vi "Read Time Out (SubVI).vi"(8 "error in (no error)":errorcluster, 9 "Time Out (ms)":u32=1000, 11 "DIO Reference":T1) -> (0 "Error Out":errorcluster, 3 "DIO Ref Out":T1)   [LabVIEW 2013]
uses:
  <vilib>/myRIO/Instrument Drivers/Onboard IO/DIO/typedefs/DIO Reference.ctl
  <vilib>/myRIO/Common/Instrument Driver Framework/Utilities/typedefs/myRIO Generic Hardware Reference.ctl
  <vilib>/myRIO/Common/Instrument Driver Framework/Utilities/typedefs/Hardware Version Enum.ctl
  <vilib>/myRIO/Common/Instrument Driver Framework/Utilities/typedefs/myRIO v1.0 Reference.ctl
  <vilib>/myRIO/Common/Instrument Driver Framework/Utilities/typedefs/Generic FPGA Reference.ctl
  <vilib>/myRIO/Common/Instrument Driver Framework/myRIO v1.0/DIO/typedefs/DIO Channels List.ctl
  <vilib>/myRIO/Common/Instrument Driver Framework/myRIO v1.0/DIO/typedefs/DIO Channels Enum.ctl
  TimeOutError.ctl
  <vilib>/Utility/error.llb/Error Cluster From Error Code.vi
  <vilib>/myRIO/Common/Instrument Driver Framework/myRIO v1.0/DIO/vis/myRIO v1.0 Read DIO.vi
  <vilib>/myRIO/Instrument Drivers/Onboard IO/DIO/DIO.lvlib
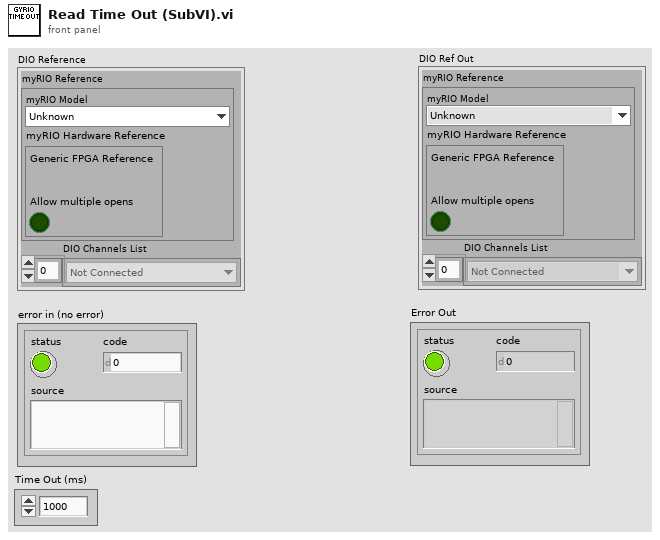
[diagram p1: front panel]
types:
  T1 = typedef "DIO.lvlib/DIO Reference.ctl" = cluster{"myRIO Reference":T2, "DIO Channels List":T6}
  T2 = typedef "myRIO Generic Hardware Reference.ctl" = cluster{"myRIO Model":T3, "myRIO Hardware Reference":T4}
  T3 = typedef "Hardware Version Enum.ctl" = enum16{"Unknown", "myRIO-1900", "myRIO-1950"}
  T4 = typedef "myRIO v1.0 Reference.ctl" = cluster{"Generic FPGA Reference":T5, "Allow multiple opens":bool}
  T5 = typedef "Generic FPGA Reference.ctl" = refnum<k20>
  T6 = typedef "DIO Channels List.ctl" = T7[]
  T7 = typedef "DIO Channels Enum.ctl" = enum16{"Not Connected", "C/DIO0", "C/DIO1", "C/DIO2", "C/DIO3", "C/DIO4", "C/DIO5", "C/DIO6", "C/DIO7", "A/DIO0", "A/DIO1", "A/DIO2", "A/DIO3", "A/DIO4", "A/DIO5", "A/DIO6", "A/DIO7", "A/DIO8", "A/DIO9", "A/DIO10", "A/DIO11", "A/DIO12", "A/DIO13", "A/DIO14", "A/DIO15", "B/DIO0", "B/DIO1", "B/DIO2", "B/DIO3", "B/DIO4", "B/DIO5", "B/DIO6", "B/DIO7", "B/DIO8", "B/DIO9", "B/DIO10", "B/DIO11", "B/DIO12", "B/DIO13", "B/DIO14", "B/DIO15", "LED0", "LED1", "LED2", "LED3", "Button0"}
  T8 = typedef "TimeOutError.ctl" = errorcluster
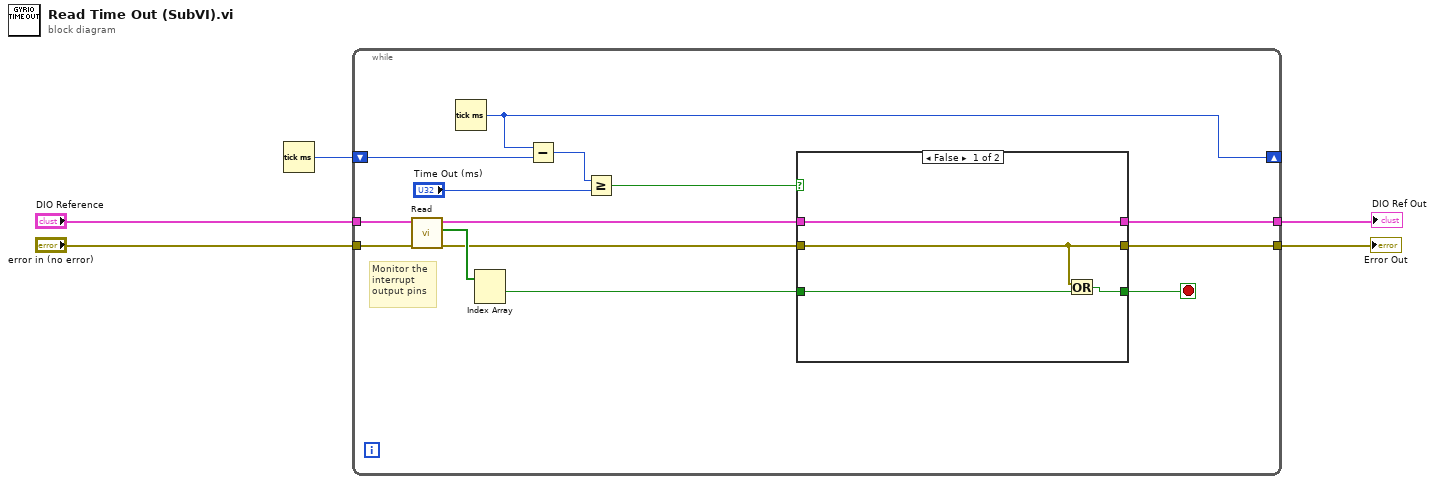
[diagram p0: block diagram]
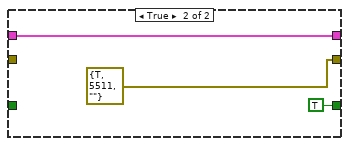
[diagram p2: hidden frame]
diagram:
  n1 = Tick Count (ms)() -> (millisecond timer value=w1:u32)
  n2 = while {
    tunnel: "error in (no error)" -> [w18]
    tunnel: "DIO Reference" -> [w17]
    tunnel: [w6] -> w2
    tunnel: [w7] -> w3
    shift-right: [w10] -> _
    shift-left: w1 -> [w13]
    stop <- w15 stop-if-true
    # "Monitor the\ninterrupt\noutput pins"
    n3 = call <vilib>:"Read.vi"("error in (no error)"=w18, "DIO Ref In"=w17) -> ("error out"=w14:errorcluster, "Values"=w19:bool[], "DIO Ref Out"=w8:T1)  [unwired: 7 in]
    n4 = Tick Count (ms)() -> (millisecond timer value=w10:u32)
    n5 = Index Array "Index Array"(array=w19) -> (element #1=w16:bool)  [unwired: 2 in, 1 out]
    n6 = Subtract(x=w10, y=w13) -> (x-y=w12:u32)
    n7 = Greater Or Equal?(x=w12, y="Time Out (ms)") -> (x >= y?=w9:bool)
    n8 = case shown="False" w9 {
      tunnel: w16 -> [w23 _]
      tunnel: [w22 TRUE] -> w15
      tunnel: w14 -> [w20 _]
      tunnel: w8 -> [w21 w25]
      tunnel: [w21 w25] -> w7
      tunnel: [w20 T8 {"status"=TRUE, "code"=5511, "source"=""} ("error constant")] -> w6
      frame False {
        n9 = Or(x=w20, y=w23) -> (x .or. y?=w22:bool)
      }
      frame True {
      }
    }
  }
  "Error Out" <- w2
  "DIO Ref Out" <- w3
